vi "DiffIO State.vi"(9 "FIFO Indexes":T2, 10 "Diff I/O In":T1, 11 "Device Outputs in":dbl[](array[numeric])) -> (3 "Device Outputs out":dbl[](array[numeric]))   [LabVIEW 2015, in "DCM Engine.lvlib"]
uses:
  DCM Engine.lvlib
  <vilib>/Powertrain Controls/Device Drivers/DCM/Tools/FPGA/8 Channels.ctl
  <vilib>/Powertrain Controls/Device Drivers/DCM/Tools/FPGA/DCM - FPGA - Tools.lvlib
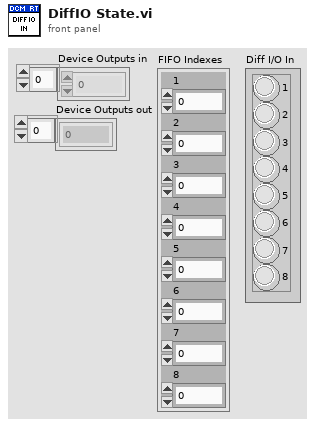
[diagram p1: front panel]
types:
  T1 = typedef "DCM - FPGA - Tools.lvlib/8 Channels.ctl" = cluster{"1":bool, "2":bool, "3":bool, "4":bool, "5":bool, "6":bool, "7":bool, "8":bool}
  T2 = cluster{"1":i32, "2":i32, "3":i32, "4":i32, "5":i32, "6":i32, "7":i32, "8":i32}
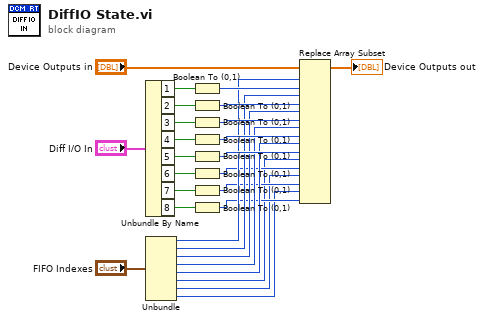
[diagram p0: block diagram]
diagram:
  n1 = Unbundle By Name("Diff I/O In") -> ("1"=w22:bool, "2"=w26:bool, "3"=w25:bool, "4"=w24:bool, "5"=w23:bool, "6"=w9:bool, "7"=w8:bool, "8"=w7:bool)
  n2 = Unbundle("FIFO Indexes") -> ("1"=w16:i32, "2"=w15:i32, "3"=w14:i32, "4"=w13:i32, "5"=w12:i32, "6"=w3:i32, "7"=w2:i32, "8"=w1:i32)
  n3 = Boolean To (0,1)(Boolean=w22) -> (0, 1=w21:i16)
  n4 = Boolean To (0,1)(Boolean=w26) -> (0, 1=w20:i16)
  n5 = Boolean To (0,1)(Boolean=w25) -> (0, 1=w19:i16)
  n6 = Boolean To (0,1)(Boolean=w24) -> (0, 1=w17:i16)
  n7 = Boolean To (0,1)(Boolean=w23) -> (0, 1=w18:i16)
  n8 = Boolean To (0,1)(Boolean=w9) -> (0, 1=w6:i16)
  n9 = Boolean To (0,1)(Boolean=w8) -> (0, 1=w5:i16)
  n10 = Boolean To (0,1)(Boolean=w7) -> (0, 1=w4:i16)
  n11 = Replace Array Subset(array="Device Outputs in", new element #1=w21, index #1=w16, new element #2=w20, index #2=w15, new element #3=w19, index #3=w14, new element #4=w17, index #4=w13, new element #5=w18, index #5=w12, new element #6=w6, index #6=w3, new element #7=w5, index #7=w2, new element #8=w4, index #8=w1) -> (→"Device Outputs out":dbl[])
